vi "SR201_test.vi"() -> ()   [LabVIEW 2019]
panel:
  in  "port":u16=6722
  in  "address":string="192.168.24.184"
  out "bits_set":i32
  out "ch_2_out":bool
  out "ch_1_out":bool
  out "ch_2_set":bool
  out "ch_1_set":bool
  out "time":timestamp format="%<%Y-%m-%d %H:%M:%S>T"
  out "status":bool
  in  "wait (ms)":u32=1000
  in  "stop":bool
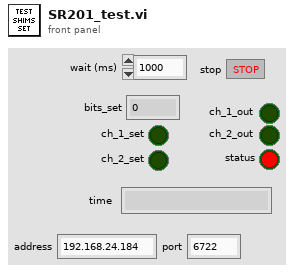
[diagram p1: front panel]
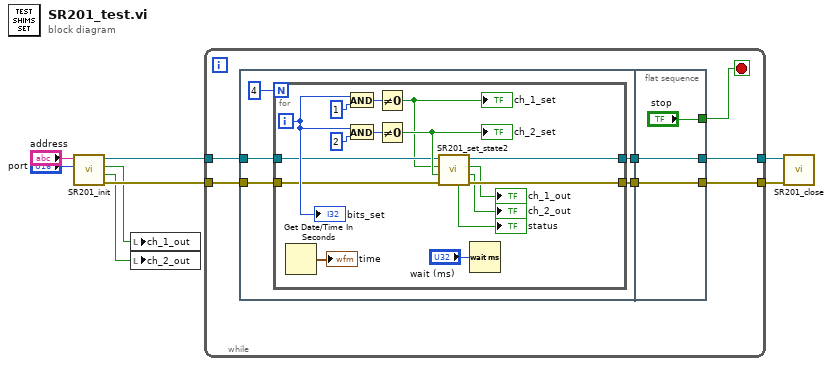
[diagram p0: block diagram]
diagram:
  n1 = call "SR201_init.vi"("port"="port", "address"="address") -> ("error out"=w6:errorcluster, "ch2"=w1:bool, "ch1"=w2:bool, "conn_id"=w8:refnum<k5>)  [unwired: 5 in, 1 out]
  n2 = local write "ch_1_out"(w2) -> ()
  n3 = local write "ch_2_out"(w1) -> ()
  n4 = while {
    tunnel: w8 -> [w14]
    tunnel: [w12] -> w7
    tunnel: w6 -> [w11]
    tunnel: [w9] -> w5
    stop <- w15 stop-if-true
    n5 = flat-sequence {
      tunnel: w14 -> [w19]
      tunnel: [w18] -> w13
      tunnel: w11 -> [w17]
      tunnel: [w16] -> w10
      tunnel: ["stop"] -> w15
      tunnel: w13 -> [w38]
      tunnel: [w38] -> w12
      tunnel: w10 -> [w37]
      tunnel: [w37] -> w9
      frame #0 {
        n6 = for {
          N: 4 -> [_]
          tunnel: w19 -> [w23]
          tunnel: [w28] -> w18
          tunnel: w17 -> [w22]
          tunnel: [w27] -> w16
          i -> [w30]
          n7 = Get Date/Time In Seconds() -> (seconds since 1Jan1904=→"time":timestamp)
          n8 = And(x=w30, y=u32 1) -> (x .and. y?=w33:u32)
          n9 = And(x=w30, y=u32 2) -> (x .and. y?=w31:u32)
          n10 = Not Equal To 0?(x=w33) -> (x != 0?=w21:bool)
          "ch_1_set" <- w21
          n11 = Not Equal To 0?(x=w31) -> (x != 0?=w24:bool)
          "ch_2_set" <- w24
          n12 = call "SR201_set_state2.vi"("error in"=w22, "state_ch2"=w24, "state_ch1"=w21, "conn_id_in"=w23) -> ("error out"=w27:errorcluster, "ch2"=→"ch_2_out":bool, "ch1"=→"ch_1_out":bool, "conn_id_out"=w28:refnum<k5>, "status"=→"status":bool)  [unwired: 2 in, 1 out]
          n13 = Wait (ms)(milliseconds to wait="wait (ms)") -> ()  [unwired: 1 out]
          "bits_set" <- w30
        }
      }
      frame #1 {
      }
    }
  }
  n14 = call "SR201_close.vi"("error in"=w5, "conn_id"=w7) -> ()  [unwired: 8 in, 2 out]
